vi "New VISA TCP Listener.vi"(8 "error in (no error)":errorcluster) -> (0 "error out":errorcluster, 3 "VISA TCP Listener out":refnum<class "VISA TCP Listener.lvclass">)   [LabVIEW 2013, in "Sockets.lvlib" / "VISA TCP Listener.lvclass"]
uses:
  VISA TCP Listener.lvclass
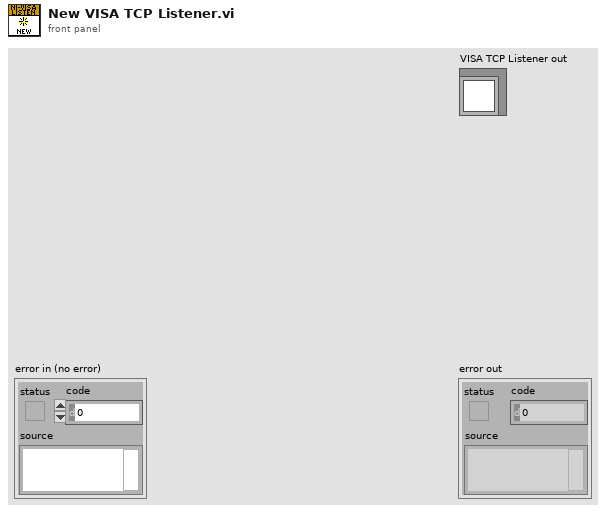
[diagram p1: front panel]
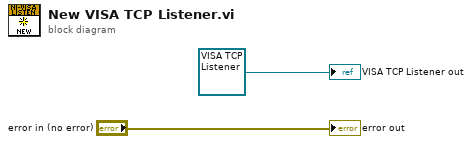
[diagram p0: block diagram]
diagram:
  "error out" <- "error in (no error)"
  "VISA TCP Listener out" <- refnum<class "VISA TCP Listener.lvclass"> refnum ("VISA TCP Listener in")
